vi "读RFID数据.vi"(2 "初始化串口":bool=TRUE caption="写入", 3 "VISA resource name out 2":refnum<visa-resource-name>) -> (0 "读取数据":string, 1 "VISA resource name out":refnum<visa-resource-name>)   [LabVIEW 2011]
panel:
  in  "节点地址":i16=2
  out "UID":string
  out "命令码":string
  out "read buffer":string
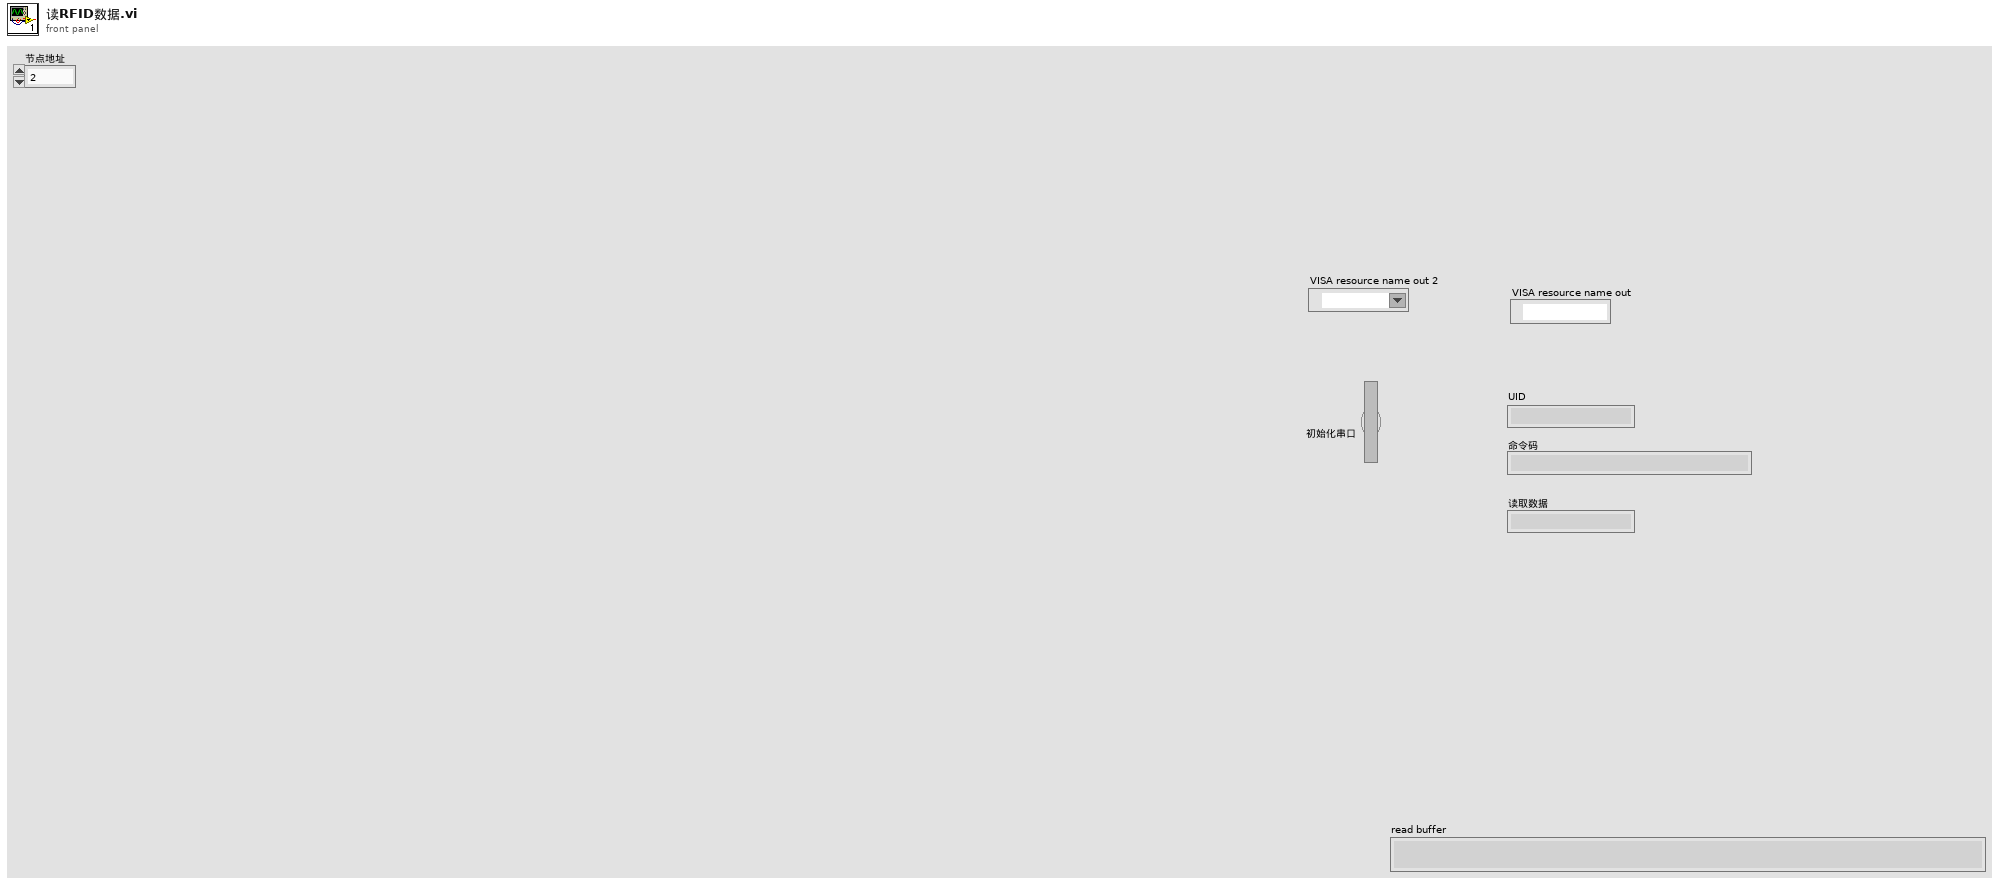
[diagram p1: front panel]
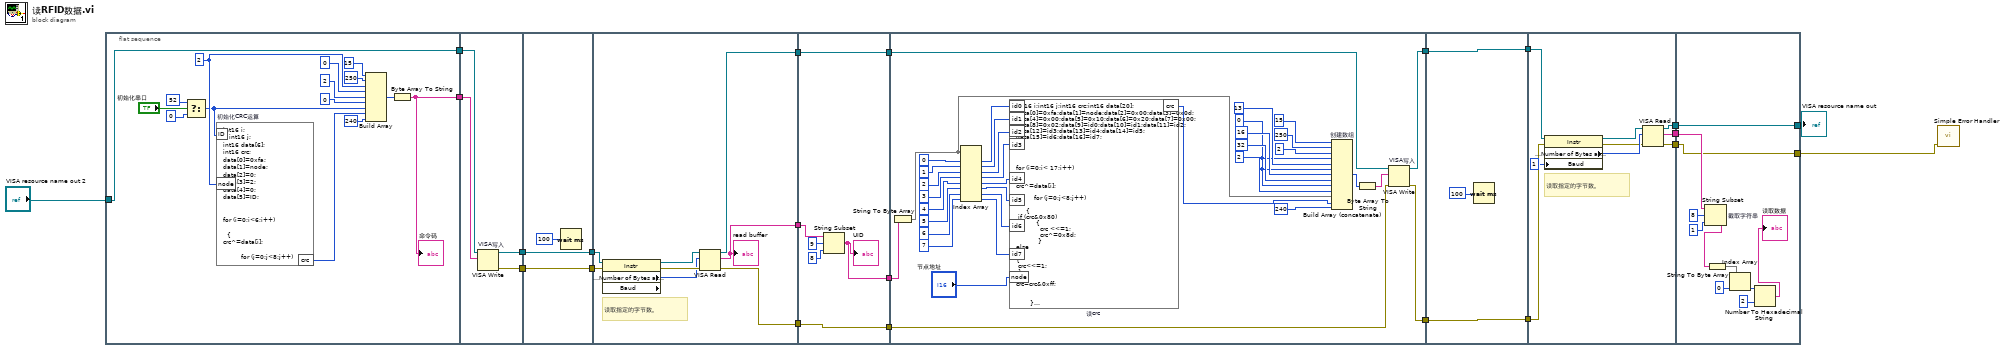
[diagram p0: block diagram]
diagram:
  n1 = flat-sequence {
    tunnel: [w23] -> w22
    tunnel: [w24] -> w21
    tunnel: "VISA resource name out 2" -> [w23]
    tunnel: w22 -> [w38]
    tunnel: [w41] -> w20
    tunnel: [w40] -> w19
    tunnel: w21 -> [w39]
    tunnel: w20 -> [w43]
    tunnel: [w43] -> w18
    tunnel: w19 -> [w42]
    tunnel: [w42] -> w17
    tunnel: w18 -> [w50]
    tunnel: w17 -> [w49]
    tunnel: [w47] -> w16
    tunnel: [w46] -> w15
    tunnel: [w45] -> w14
    tunnel: w16 -> [w56]
    tunnel: w15 -> [w54]
    tunnel: [w55] -> w13
    tunnel: [w54] -> w11
    tunnel: [w53] -> w12
    tunnel: w14 -> [w53]
    tunnel: w13 -> [w67]
    tunnel: w12 -> [w64]
    tunnel: w11 -> [w63]
    tunnel: [w60] -> w10
    tunnel: [w59] -> w9
    tunnel: w10 -> [w95]
    tunnel: [w95] -> w8
    tunnel: w9 -> [w94]
    tunnel: [w94] -> w7
    tunnel: w8 -> [w102]
    tunnel: w7 -> [w101]
    tunnel: [w100] -> w6
    tunnel: [w99] -> w5
    tunnel: [w98] -> w4
    tunnel: w6 -> [w114]
    tunnel: w5 -> [w113]
    tunnel: w4 -> [w112]
    tunnel: [w113] -> w2
    tunnel: [w112] -> w3
    frame #0 {
      w37 = i16 2 ("节点地址")
      n2 = Select(t=52, s="初始化串口", f=0) -> (s? t:f=w26:i32)
      n3 = formula code="int16 i;\n   int16 j;\nint16 data[6];\nint16 crc;\ndata[0]=0xfa;\ndata[1]=node;\ndata[2]=0;\ndata[3]=2;\ndata[4]=0;\ndata[5]=ID;\n\n\nfor (i=0;i<6;i++)\n\n  {\ncrc^=data[i];\n\n         for (j=0;j<8;j++)\n\n     { \n if (crc&0x80)\n          {\n            crc <<=1;\n            crc^=0x8d;\n           }\nelse\n    \n{\n\tcrc<<=1;\n\t}\n\ncrc=crc&0xff;\n\n\n       }\n\n}" "初始化CRC运算"("node"=w37, "ID"=w26) -> ("crc"=w25:i16)
      n4 = Build Array(i16 15 ("数组"), i16 250 ("数组"), w37, i16 0 ("数组"), i16 2 ("数组"), i16 0 ("数组"), w26, w25, i16 240 ("数组")) -> (w36:i32[])
      n5 = Byte Array To String(unsigned byte array=w36) -> (string=w24:string)
      "命令码" <- w24
    }
    frame #1 {
      n6 = VISA Write "VISA写入"(VISA resource name=w38, write buffer=w39) -> (VISA resource name out=w41:refnum<visa-resource-name>, error out=w40:errorcluster)  [unwired: 1 in, 1 out]
    }
    frame #2 {
      n7 = Wait (ms)(milliseconds to wait=u32 100 ("等待时间（毫秒）")) -> ()  [unwired: 1 out]
    }
    frame #3 {
      # "读取指定的字节数。"
      n8 = property class="Instr" props=["Serial Settings:Number of Bytes at Serial Port", "Baud"](reference=w50, error in=w49) -> (reference out=w51:refnum<visa-resource-name>, error out=w52:errorcluster, "Serial Settings:Number of Bytes at Serial Port"=w48:u32)  [unwired: 1 out]
      n9 = VISA Read(VISA resource name=w51, byte count=w48, error in (no error)=w52) -> (VISA resource name out=w45:refnum<visa-resource-name>, read buffer=w47:string, error out=w46:errorcluster)  [unwired: 1 out]
      "read buffer" <- w47
    }
    frame #4 {
      n10 = String Subset(string=w56, offset (0)=9 ("偏移量(0)"), length (rest)=8 ("长度（剩余）")) -> (substring=w55:string)
      "UID" <- w55
    }
    frame #5 {
      w87 = i16 0 ("数组")
      n11 = String To Byte Array(string=w67) -> (unsigned byte array=w66:u8[])
      n12 = Index Array(array=w66, index #1=0 ("索引"), index #2=1 ("索引"), index #3=2 ("索引"), index #4=3 ("索引"), index #5=4 ("索引"), index #6=5 ("索引"), index #7=6 ("索引"), index #8=7 ("索引")) -> (element #1=w76:u8, element #2=w77:u8, element #3=w78:u8, element #4=w79:u8, element #5=w80:u8, element #6=w81:u8, element #7=w82:u8, element #8=w83:u8)
      n13 = formula code="int16 i;int16 j;int16 crc;int16 data[20];\ndata[0]=0xfa;data[1]=node;data[2]=0x00;data[3]=0x0d;\ndata[4]=0x00;data[5]=0x10;data[6]=0x20;data[7]=0x00;\ndata[8]=0x02;data[9]=id0;data[10]=id1;data[11]=id2;\ndata[12]=id3;data[13]=id4;data[14]=id5;\ndata[15]=id6;data[16]=id7;\n\n\n\n\nfor (i=0;i< 17;i++)\n\n  {\ncrc^=data[i];\n\n         for (j=0;j<8;j++)\n\n     { \n if (crc&0x80)\n          {\n            crc <<=1;\n            crc^=0x8d;\n           }\nelse\n    \n{\n\tcrc<<=1;\n\t}\n\ncrc=crc&0xff;\n\n\n       }\n\n}" "读crc"("node"="节点地址", "id0"=w76, "id1"=w77, "id2"=w78, "id3"=w79, "id4"=w80, "id5"=w81, "id6"=w82, "id7"=w83) -> ("crc"=w65:i16)
      n14 = Build Array (concatenate) "创建数组"(i16 15 ("数组"), i16 250 ("数组"), i16 2 ("数组"), w87, i16 13 ("数组"), w87, i16 16 ("数组"), i16 32 ("数组"), w87, i16 2 ("数组"), w66, w65, i16 240 ("数组")) -> (w62:i16[])
      n15 = Byte Array To String(unsigned byte array=w62) -> (string=w61:string)
      n16 = VISA Write "VISA写入"(VISA resource name=w64, write buffer=w61, error in (no error)=w63) -> (VISA resource name out=w60:refnum<visa-resource-name>, error out=w59:errorcluster)  [unwired: 1 out]
    }
    frame #6 {
      n17 = Wait (ms)(milliseconds to wait=u32 100 ("等待时间（毫秒）")) -> ()  [unwired: 1 out]
    }
    frame #7 {
      # "读取指定的字节数。"
      n18 = property class="Instr"(reference=w102, error in=w101, "Baud"=u32 1 ("Serial Settings:Baud Rate")) -> (reference out=w104:refnum<visa-resource-name>, error out=w103:errorcluster, "Serial Settings:Number of Bytes at Serial Port"=w105:u32)
      n19 = VISA Read(VISA resource name=w104, byte count=w105, error in (no error)=w103) -> (VISA resource name out=w99:refnum<visa-resource-name>, read buffer=w100:string, error out=w98:errorcluster)  [unwired: 1 out]
    }
    frame #8 {
      n20 = String Subset "截取字符串"(string=w114, offset (0)=8 ("偏移量(0)"), length (rest)=1 ("长度（剩余）")) -> (substring=w109:string)
      n21 = String To Byte Array(string=w109) -> (unsigned byte array=w108:u8[])
      n22 = Index Array(array=w108, index=0 ("索引")) -> (element=w111:u8)
      n23 = Number To Hexadecimal String(1:i16 2 ("宽度(-)"), 2:w111) -> (0:→"读取数据":string)
    }
  }
  n24 = call <vilib>:"Simple Error Handler.vi"("error in (no error)"=w3) -> ()  [unwired: 1 in, 8 out]
  "VISA resource name out" <- w2
